vi "T1_viewer_gui.vi"() -> ()   [LabVIEW 2014]
uses:
  <vilib>/Analysis/NI_AALBase.lvlib
panel:
  in  "plots_tabs":enum32{"T1 curves", "Pulses", "Overlap pulses"}(tab)
  out "t1_curves":T1(graph)
  out "detections":u32[](graph)
  out "detections_norm":dbl[](graph)
  out "pulses":u32[][](graph)
  in  "show_all":bool
  in  "hide_all":bool
  out "snr_pulses":dbl
  out "mean_pulses":dbl format="%0.2f"
  in  "normalise_method":enum16{"No normalise", "Minimum", "Same pulse"}(ring)
  in  "save":bool
  in  "parameters":enum32{"No Selection", "uniform", "proposed"}(radio)=enum."uniform" caption="Parameters"
  in  "use_proposed_correction":bool
  in  "propose_rw":bool
  in  "propose_correction":bool
  in  "calc_parameters":bool
  in  "read_width_us":dbl
  in  "correction_us":dbl
  in  "compute_T1":bool
  in  "parameters":i32(listbox)
  out "progress":u8(slide) scale=0.0..100.0
  in  "plot_curves":bool
  in  "file_list":i32[](listbox)
  in  "files_folder":path
  in  "stop":bool
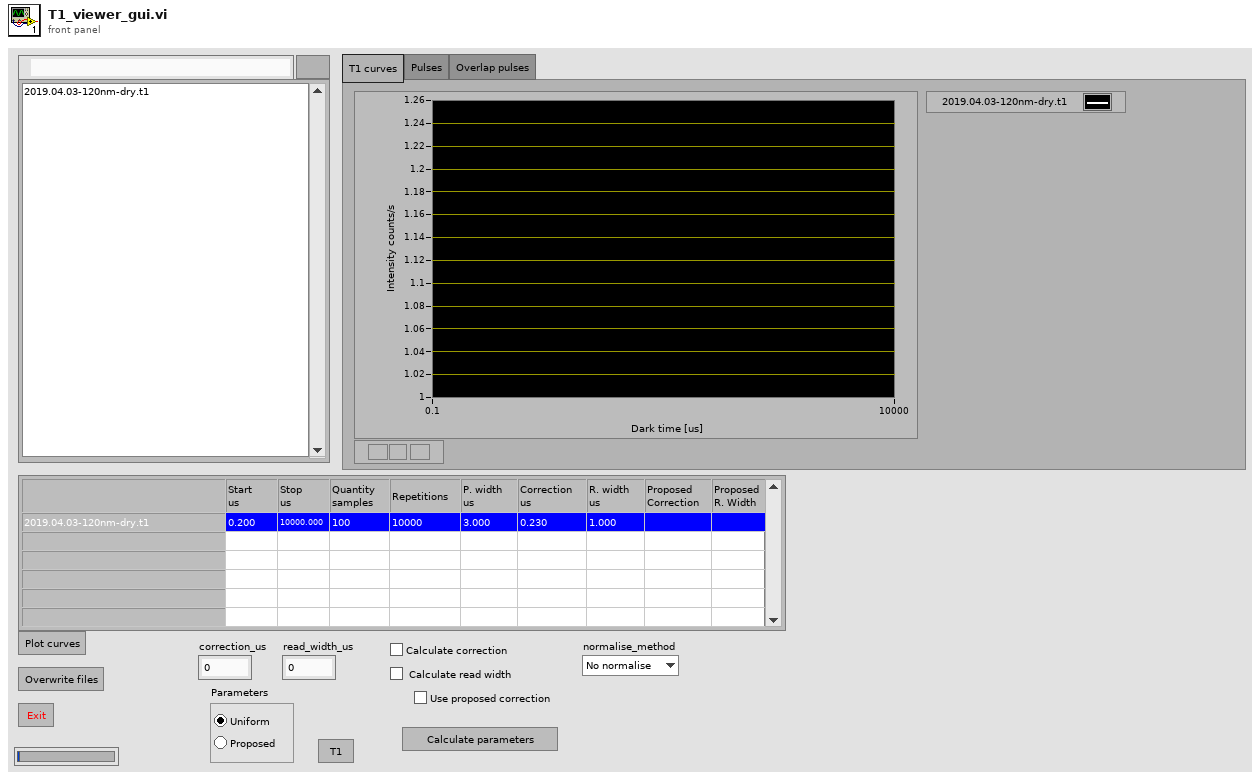
[diagram p1: front panel]
types:
  T1 = cluster{"dark_times_us":dbl[], "measured_signal":dbl[]}[]
  T2 = cluster{"dark_time_us":dbl[], "PL_signal":dbl[]}[]
  T3 = enum16{"standby", "plot", "fit", "compute_T1", "calc_correction"}
  T4 = enum16{"standby", "plot", "fit", "compute_T1", "calc_correction", "save"}
  T5 = enum16{"standby", "plot", "fit", "compute_T1", "calc_correction", "save", "plot_pulses"}
  T6 = cluster{"dark_times_us":dbl[], "measured_signal":dbl[]}
  T7 = cluster{"dark_times_us":dbl[], "pulse_width_us":dbl, "read_delay_us":dbl, "read_width_us":dbl, "repetitions":i32, "sampling_mode":enum16{"Normal", "Sweep"}, "correction_us":dbl}
  T8 = cluster{"dark_times":dbl[], "fitted_signal":dbl[]}
  T9 = cluster{"Ie":dbl, "Cm":dbl, "Tm":dbl, "C1":dbl, "T1":dbl, "mse":dbl}
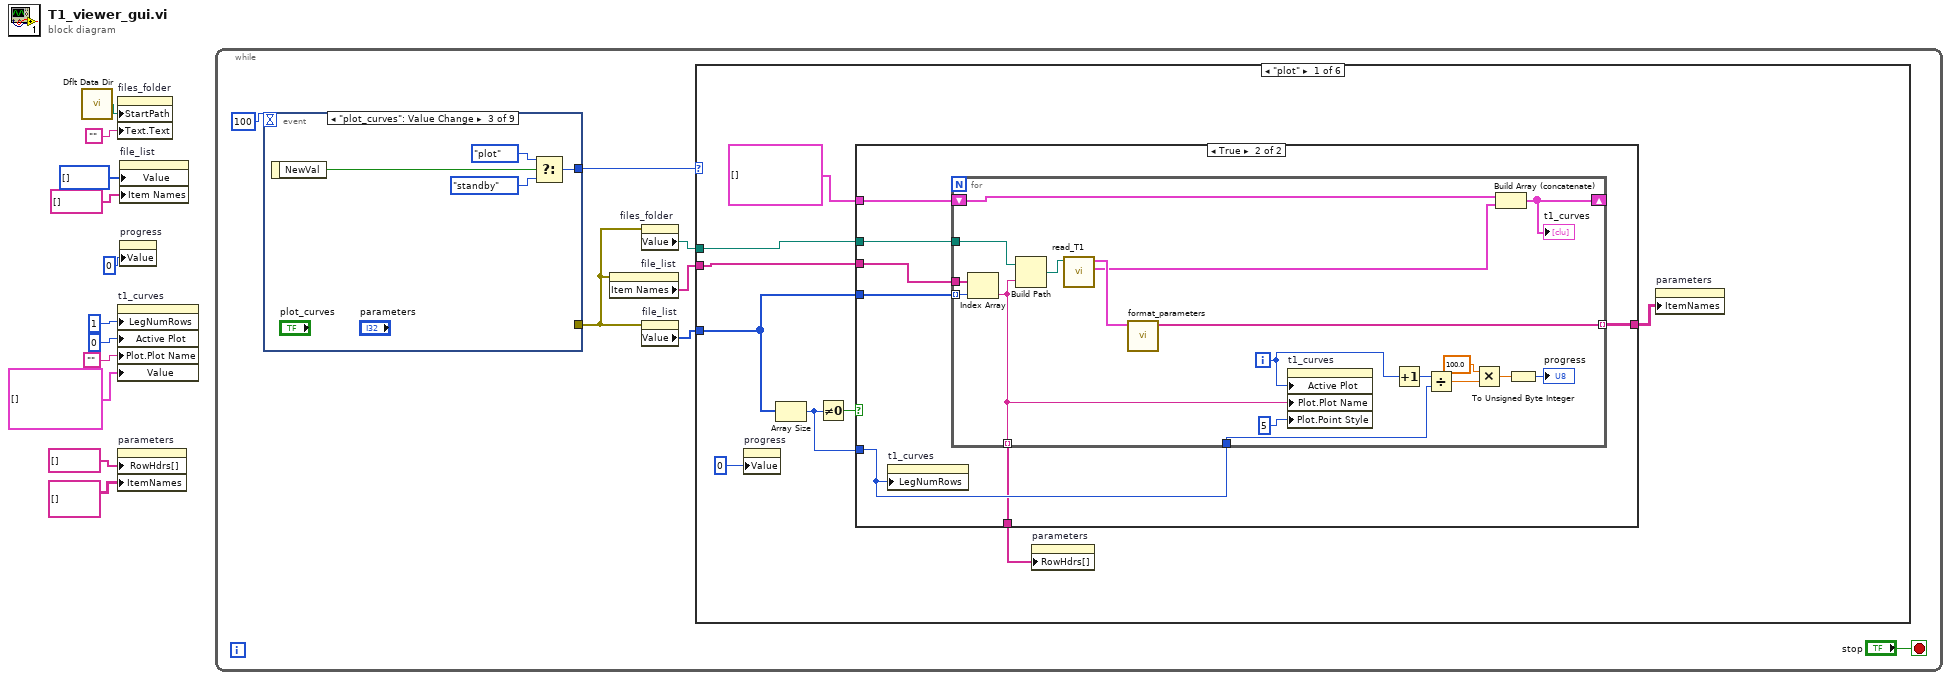
[diagram p0: block diagram]
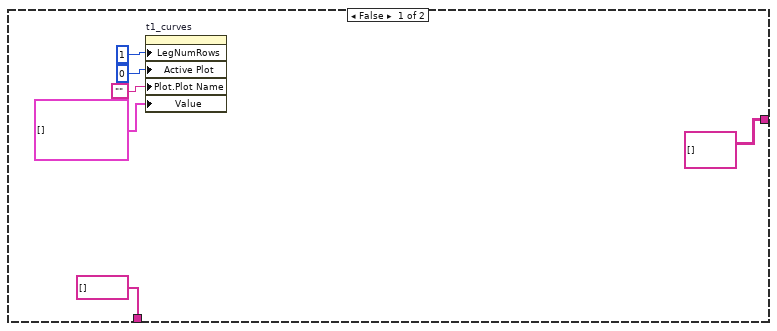
[diagram p2: hidden frame]
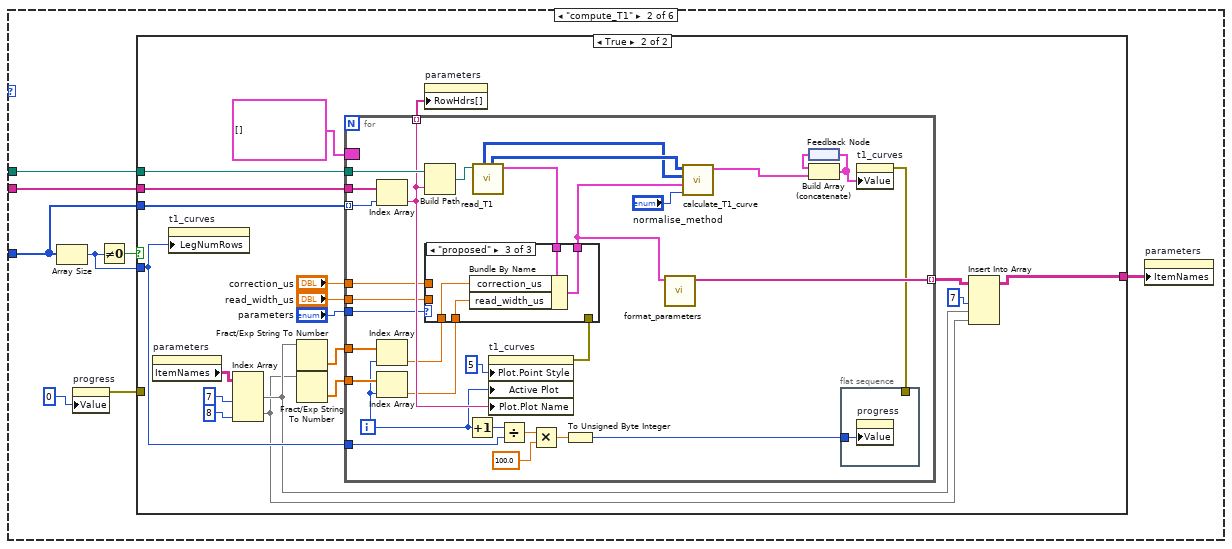
[diagram p3: hidden frame]
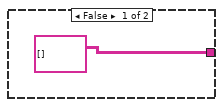
[diagram p4: hidden frame]
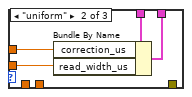
[diagram p6: hidden frame]
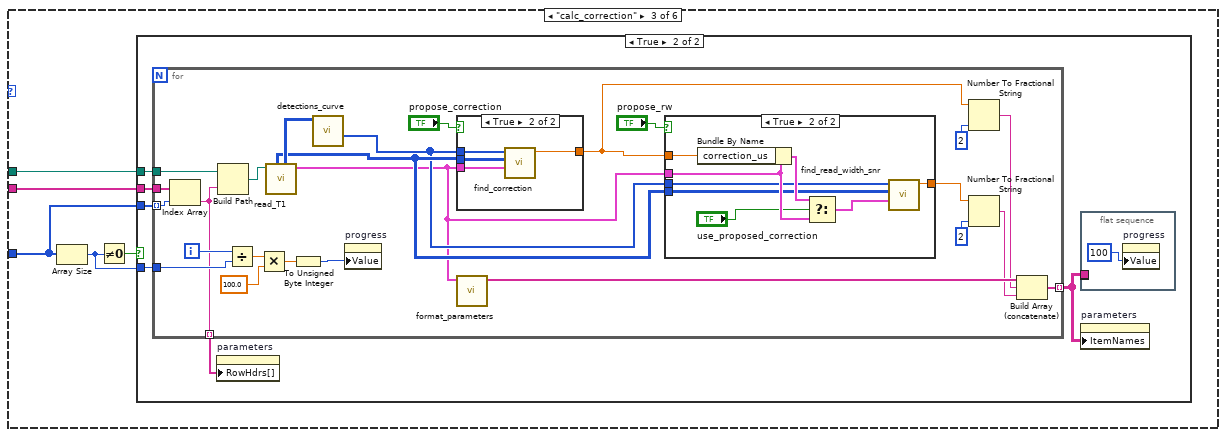
[diagram p7: hidden frame]
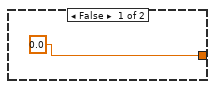
[diagram p9: hidden frame]
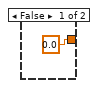
[diagram p10: hidden frame]
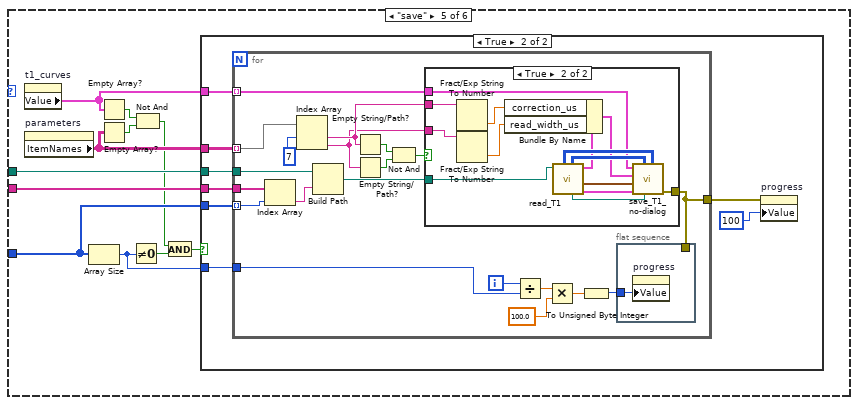
[diagram p12: hidden frame]
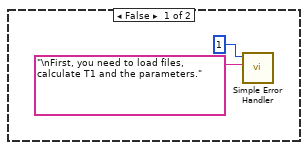
[diagram p13: hidden frame]
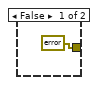
[diagram p14: hidden frame]
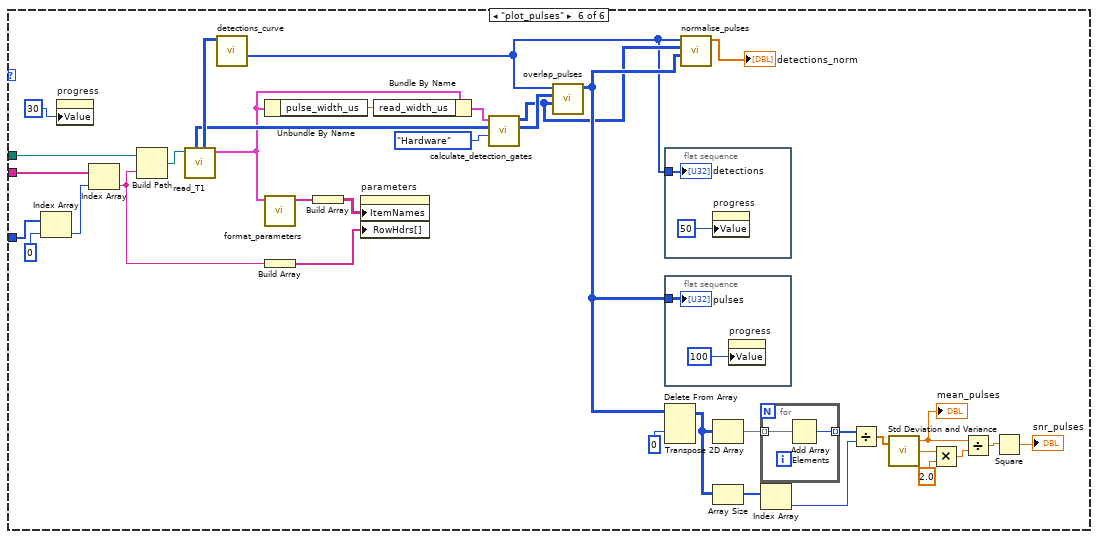
[diagram p15: hidden frame]
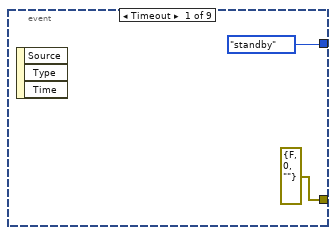
[diagram p16: hidden frame]
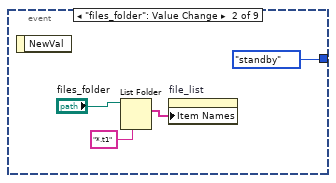
[diagram p17: hidden frame]
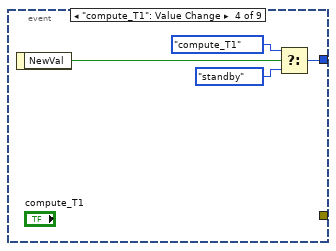
[diagram p18: hidden frame]
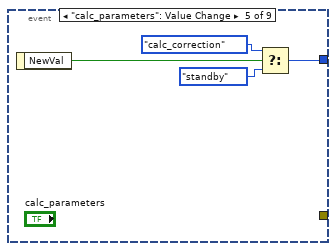
[diagram p19: hidden frame]
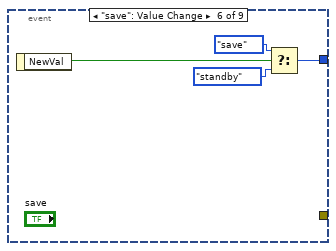
[diagram p20: hidden frame]
diagram:
  n1 = call <vilib>:"Dflt Data Dir.vi"() -> ("App:Default Data Directory"=w9:path)
  n2 = property on="files_folder" class="Path"("StartPath"=w9, "Text.Text"="") -> ()  [unwired: 2 in, 2 out]
  n3 = property on="t1_curves" class="XYGraph (strict)"("LegNumRows"=u32 1 ("Legend:Number of Rows"), "Active Plot"=u32 0, "Plot.Plot Name"="", "Value"=T1 [] ("t1_curves")) -> ()  [unwired: 2 in, 2 out]
  n4 = property on="parameters" class="MCListbox (strict)"("RowHdrs[]"=string[] [] ("Row Header Strings[]"), "ItemNames"=string[][] [] ("Item Names")) -> ()  [unwired: 2 in, 2 out]
  n5 = property on="file_list" class="LstBox (strict)"("Value"=i32[] [] ("file_list"), "Item Names"=string[] []) -> ()  [unwired: 2 in, 2 out]
  n6 = property on="progress" class="Slide (strict)"("Value"=u8 0 ("progress")) -> ()  [unwired: 2 in, 2 out]
  n7 = while {
    stop <- "stop" stop-if-true
    n8 = event shown="[2] \"plot_curves\": Value Change" {
      selector: _ -> [_ _ _ _ _ _ _ _ _]
      dyn-events: _ -> [_ _ _ _ _ _ _ _ _]
      timeout: 100 -> [_ _ _ _ _ _ _ _ _]
      tunnel: [enum16{"standby", "plot"}."standby" enum16{"standby", "plot"}."standby" w286 w291 w294 w298 T5."standby" T5."standby" w311] -> w16
      tunnel: [errorcluster {"status"=FALSE, "code"=0, "source"=""} ("error in (no error)") _ _ _ _ _ _ _ _] -> w12
      event Timeout {
        n9 = event-data() -> ()  [unwired: 1 in, 3 out]
      }
      event "files_folder": Value Change {
        n10 = event-data() -> ()  [unwired: 1 in, 1 out]
        n11 = List Folder(path="files_folder", pattern="*.t1") -> (filenames=w281:string[])  [unwired: 2 in, 3 out]
        n12 = property on="file_list" class="LstBox (strict)"("Item Names"=w281) -> ()  [unwired: 2 in, 2 out]
      }
      event "plot_curves": Value Change {
        n13 = event-data() -> ("NewVal"=w287:bool)  [unwired: 1 in]
        n14 = Select(t=enum16{"standby", "plot", "fit"}."plot", s=w287, f=enum16{"standby", "plot", "fit"}."standby") -> (s? t:f=w286:enum16{"standby", "plot", "fit"})
      }
      event "compute_T1": Value Change {
        n15 = event-data() -> ("NewVal"=w288:bool)  [unwired: 1 in]
        n16 = Select(t=enum16{"standby", "plot", "fit", "compute_T1"}."compute_T1", s=w288, f=enum16{"standby", "plot", "fit", "compute_T1"}."standby") -> (s? t:f=w291:enum16{"standby", "plot", "fit", "compute_T1"})
      }
      event "calc_parameters": Value Change {
        n17 = event-data() -> ("NewVal"=w292:bool)  [unwired: 1 in]
        n18 = Select(t=T3."calc_correction", s=w292, f=T3."standby") -> (s? t:f=w294:T3)
      }
      event "save": Value Change {
        n19 = event-data() -> ("NewVal"=w296:bool)  [unwired: 1 in]
        n20 = Select(t=T4."save", s=w296, f=T4."standby") -> (s? t:f=w298:T4)
      }
      event "hide_all": Value Change {
        n21 = event-data() -> ()  [unwired: 1 in, 1 out]
        n22 = while {
          i -> [w303]
          stop <- w301 stop-if-true
          n23 = property on="pulses" class="WFGraph (strict)"("Active Plot"=w303, "Plot.Visible?"=FALSE ("Plot.Visible")) -> (error out=w301:errorcluster)  [unwired: 2 in, 1 out]
        }
      }
      event "show_all": Value Change {
        n24 = event-data() -> ()  [unwired: 1 in, 1 out]
        n25 = while {
          i -> [w306]
          stop <- w307 stop-if-true
          n26 = property on="pulses" class="WFGraph (strict)"("Active Plot"=w306, "Plot.Visible?"=TRUE ("Plot.Visible")) -> (error out=w307:errorcluster)  [unwired: 2 in, 1 out]
        }
      }
      event "file_list": Value Change {
        n27 = event-data() -> ("NewVal"=w310:i32[])  [unwired: 1 in]
        n28 = Empty Array?(array=w310) -> (empty?=w309:bool)
        n29 = Not(x=w309) -> (.not. x?=w308:bool)
        n30 = case shown="True" w308 {
          tunnel: [T5."standby" w313] -> w311
          frame False {
          }
          frame True {
            n31 = case shown="\"T1 curves\", Default" "plots_tabs" {
              tunnel: [T5."standby" T5."plot_pulses" T5."plot_pulses"] -> w313
              frame "T1 curves", Default {
              }
              frame "Pulses" {
              }
              frame "Overlap pulses" {
              }
            }
          }
        }
      }
    }
    n32 = property on="file_list" class="LstBox (strict)"(error in=w12) -> ("Item Names"=w14:string[])  [unwired: 1 in, 2 out]
    n33 = property on="files_folder" class="Path"(error in=w12) -> ("Value"=w15:path)  [unwired: 1 in, 2 out]
    n34 = property on="file_list" class="LstBox (strict)"(error in=w12) -> ("Value"=w13:i32[])  [unwired: 1 in, 2 out]
    n35 = case shown="\"plot\"" w16 {
      tunnel: w15 -> [w19 w65 w132 _ w190 w271]
      tunnel: w14 -> [w20 w64 w131 _ w189 w270]
      tunnel: w13 -> [w21 w62 w129 _ w188 w258]
      frame "plot" {
        n36 = property on="progress" class="Slide (strict)"("Value"=u8 0 ("progress")) -> ()  [unwired: 2 in, 2 out]
        n37 = Array Size(array=w21) -> (size(s)=w26:i32)
        n38 = Not Equal To 0?(x=w26) -> (x != 0?=w27:bool)
        n39 = case shown="True" w27 {
          tunnel: w19 -> [_ w40]
          tunnel: w21 -> [_ w39]
          tunnel: w26 -> [_ w38]
          tunnel: T1 [] ("t1_curves") -> [_ w37]
          tunnel: w20 -> [_ w36]
          tunnel: [string[] [] w35] -> w23
          tunnel: [string[][] [] ("parameters") w34] -> w22
          frame False {
            n40 = property on="t1_curves" class="XYGraph (strict)"("LegNumRows"=u32 1 ("Legend:Number of Rows"), "Active Plot"=u32 0, "Plot.Plot Name"="", "Value"=T1 [] ("t1_curves")) -> ()  [unwired: 2 in, 2 out]
          }
          frame True {
            n41 = property on="t1_curves" class="XYGraph (strict)"("LegNumRows"=w38) -> ()  [unwired: 2 in, 2 out]
            n42 = for {
              tunnel: w39 -> [w58] mode=indexing
              tunnel: w40 -> [w56]
              tunnel: w38 -> [w43]
              shift-right: [w54] -> _
              shift-left: w37 -> [w42]
              tunnel: w36 -> [w53]
              tunnel: [w52] -> w35 mode=indexing
              tunnel: [w50] -> w34 mode=indexing
              i -> [w44]
              n43 = Index Array(array=w53, index=w58) -> (element=w52:string)
              n44 = Build Path(base path=w56, name or relative path=w52) -> (appended path=w57:path)
              n45 = call "read_T1.vi"("file_path"=w57) -> ("T1_curve"=w41:T6, "T1_parameters"=w51:T7)  [unwired: 4 in, 5 out]
              n46 = call "format_parameters.vi"("T1_parameters"=w51) -> ("parameters_strg"=w50:string[])  [unwired: 9 in, 1 out]
              n47 = property on="t1_curves" class="XYGraph (strict)"("Active Plot"=w44, "Plot.Plot Name"=w52, "Plot.Point Style"=u8 5) -> ()  [unwired: 2 in, 2 out]
              n48 = Increment(x=w44) -> (x+1=w49:i32)
              n49 = Divide(x=w49, y=w43) -> (x/y=w47:dbl)
              n50 = Multiply(x=100.0, y=w47) -> (x*y=w46:dbl)
              n51 = Build Array (concatenate)(w42, w41) -> (w54:T1)
              "t1_curves" <- w54
              n52 = To Unsigned Byte Integer(number=w46) -> (unsigned 8bit integer=→"progress":u8)
            }
          }
        }
        n53 = property on="parameters" class="MCListbox (strict)"("RowHdrs[]"=w23) -> ()  [unwired: 2 in, 2 out]
        n54 = property on="parameters" class="MCListbox (strict)"("ItemNames"=w22) -> ()  [unwired: 2 in, 2 out]
      }
      frame "compute_T1" {
        n55 = Array Size(array=w62) -> (size(s)=w63:i32)
        n56 = property on="progress" class="Slide (strict)"("Value"=u8 0 ("progress")) -> (error out=w59:errorcluster)  [unwired: 2 in, 1 out]
        n57 = Not Equal To 0?(x=w63) -> (x != 0?=w66:bool)
        n58 = case shown="True" w66 {
          tunnel: w65 -> [_ w86]
          tunnel: w64 -> [_ w85]
          tunnel: w62 -> [_ w84]
          tunnel: [string[][] [] ("parameters") w75] -> w60
          tunnel: w63 -> [_ w82]
          tunnel: w59 -> [_ _]
          frame False {
          }
          frame True {
            n59 = property on="parameters" class="MCListbox (strict)"() -> ("ItemNames"=w77:string[][])  [unwired: 2 in, 2 out]
            n60 = property on="t1_curves" class="XYGraph (strict)"("LegNumRows"=w82) -> ()  [unwired: 2 in, 2 out]
            n61 = Index Array(array=w77, index (col) #1=7 ("index (row)"), index (col) #2=8 ("index (row)")) -> (element #1=w73:string[], element #2=w71:string[])  [unwired: 2 in]
            n62 = Fract/Exp String To Number(string=w73) -> (number=w72:dbl[])  [unwired: 3 in, 1 out]
            n63 = Fract/Exp String To Number(string=w71) -> (number=w70:dbl[])  [unwired: 3 in, 1 out]
            n64 = for {
              tunnel: w86 -> [w117]
              tunnel: w85 -> [w113]
              tunnel: "correction_us" -> [w97]
              tunnel: "read_width_us" -> [w96]
              border: T2 [] -> [_]
              tunnel: w84 -> [w114] mode=indexing
              tunnel: [w111] -> w76 mode=indexing
              tunnel: w82 -> [w109]
              tunnel: [w103] -> w83 mode=indexing
              tunnel: w72 -> [w94]
              tunnel: w70 -> [w92]
              tunnel: "parameters" -> [w95]
              i -> [w90]
              n65 = Index Array(array=w113, index=w114) -> (element=w103:string)
              n66 = Index Array(array=w94, index=w90) -> (element=w93:dbl)
              n67 = Index Array(array=w92, index=w90) -> (element=w91:dbl)
              n68 = Build Path(base path=w117, name or relative path=w103) -> (appended path=w116:path)
              n69 = Increment(x=w90) -> (x+1=w110:i32)
              n70 = call "read_T1.vi"("file_path"=w116) -> ("T1_parameters"=w101:T7, "timetags"=w102:u32[][], "triggers"=w100:u32[][])  [unwired: 4 in, 4 out]
              n71 = property on="t1_curves" class="XYGraph (strict)"("Plot.Point Style"=u8 5, "Active Plot"=w90, "Plot.Plot Name"=w103) -> (error out=w104:errorcluster)  [unwired: 2 in, 1 out]
              n72 = case shown="\"proposed\"" w95 {
                tunnel: [w119 w120 w127] -> w112
                tunnel: w101 -> [w119 w123 w126]
                tunnel: w96 -> [_ w122 _]
                tunnel: w97 -> [_ w121 _]
                tunnel: w104 -> [_ _ _]
                tunnel: w91 -> [_ _ w125]
                tunnel: w93 -> [_ _ w124]
                frame "No Selection", Default {
                }
                frame "uniform" {
                  n73 = Bundle By Name(cluster=w123, "correction_us"=w121, "read_width_us"=w122) -> (w120:T7)
                }
                frame "proposed" {
                  n74 = Bundle By Name(cluster=w126, "correction_us"=w124, "read_width_us"=w125) -> (w127:T7)
                }
              }
              n75 = Divide(x=w110, y=w109) -> (x/y=w108:dbl)
              n76 = Multiply(x=w108, y=100.0) -> (x*y=w106:dbl)
              n77 = To Unsigned Byte Integer(number=w106) -> (unsigned 8bit integer=w99:u8)
              n78 = call "format_parameters.vi"("T1_parameters"=w112) -> ("parameters_strg"=w111:string[])  [unwired: 9 in, 1 out]
              n79 = call "calculate_T1_curve.vi"("normalise"="normalise_method", "T1_parameters"=w112, "triggers"=w100, "timetags"=w102) -> ("T1_curve_out"=w89:cluster{"dark_time_us":dbl[], "PL_signal":dbl[]})  [unwired: 7 in]
              n80 = feedback #1() -> (w115:T2)
              n81 = Build Array (concatenate)(w115, w89) -> (w88:T2)
              n82 = feedback-in #1(w88) -> ()
              n83 = flat-sequence {
                tunnel: w99 -> [w118]
                tunnel: w98 -> [_]
                frame #0 {
                  n84 = property on="progress" class="Slide (strict)"("Value"=w118) -> ()  [unwired: 2 in, 2 out]
                }
              }
              n85 = property on="t1_curves" class="XYGraph (strict)"("Value"=w88) -> (error out=w98:errorcluster)  [unwired: 2 in, 1 out]
            }
            n86 = property on="parameters" class="MCListbox (strict)"("RowHdrs[]"=w83) -> ()  [unwired: 2 in, 2 out]
            n87 = Insert Into Array(array=w76, index (col)=7 ("disabled index (col)"), new element #1=w73, new element #2=w71) -> (w75:string[][])  [unwired: 1 in]
          }
        }
        n88 = property on="parameters" class="MCListbox (strict)"("ItemNames"=w60) -> ()  [unwired: 2 in, 2 out]
      }
      frame "calc_correction" {
        n89 = Array Size(array=w129) -> (size(s)=w128:i32)
        n90 = Not Equal To 0?(x=w128) -> (x != 0?=w130:bool)
        n91 = case shown="True" w130 {
          tunnel: w132 -> [_ w138]
          tunnel: w131 -> [_ w137]
          tunnel: w129 -> [_ w136]
          tunnel: w128 -> [_ w135]
          frame False {
          }
          frame True {
            n92 = for {
              tunnel: w138 -> [w165]
              tunnel: w137 -> [w162]
              tunnel: w136 -> [w163] mode=indexing
              tunnel: w135 -> [w161]
              tunnel: [w149] -> w133 mode=indexing
              tunnel: [w141] -> w134 mode=indexing
              i -> [w142]
              n93 = Index Array(array=w162, index=w163) -> (element=w141:string)
              n94 = Build Path(base path=w165, name or relative path=w141) -> (appended path=w164:path)
              n95 = Divide(x=w142, y=w161) -> (x/y=w160:dbl)
              n96 = Multiply(x=w160, y=100.0) -> (x*y=w158:dbl)
              n97 = call "read_T1.vi"("file_path"=w164) -> ("T1_parameters"=w151:T7, "timetags"=w156:u32[][], "triggers"=w153:u32[][])  [unwired: 4 in, 4 out]
              n98 = To Unsigned Byte Integer(number=w158) -> (unsigned 8bit integer=w157:u8)
              n99 = call "detections_curve.vi"("timetags"=w156) -> ("detections"=w152:u32[])  [unwired: 10 in]
              n100 = property on="progress" class="Slide (strict)"("Value"=w157) -> ()  [unwired: 2 in, 2 out]
              n101 = case shown="True" "propose_correction" {
                tunnel: [0.0 ("shift_us") w179] -> w148
                tunnel: w152 -> [_ w178]
                tunnel: w153 -> [_ w177]
                tunnel: w151 -> [_ w176]
                frame False {
                }
                frame True {
                  n102 = call "find_correction.vi"("T1_parameters"=w176, "triggers"=w177, "detections"=w178) -> ("shift_us"=w179:dbl)  [unwired: 8 in]
                }
              }
              n103 = call "format_parameters.vi"("T1_parameters"=w151) -> ("parameters_strg"=w150:string[])  [unwired: 9 in, 1 out]
              n104 = case shown="True" "propose_rw" {
                tunnel: [0.0 ("proposed_read_width_us") w167] -> w145
                tunnel: w151 -> [_ w172]
                tunnel: w148 -> [_ w174]
                tunnel: w153 -> [_ w169]
                tunnel: w152 -> [_ w170]
                frame False {
                }
                frame True {
                  n105 = Bundle By Name(cluster=w172, "correction_us"=w174) -> (w173:T7)
                  n106 = Select(t=w173, s="use_proposed_correction", f=w172) -> (s? t:f=w168:T7)
                  n107 = call "find_read_width_snr.vi"("T1_parameters"=w168, "triggers"=w169, "detections"=w170) -> ("read_width_us"=w167:dbl)  [unwired: 8 in]
                }
              }
              n108 = Number To Fractional String(number=w148, precision (6)=i16 2) -> (F-format string=w144:string)  [unwired: 2 in]
              n109 = Number To Fractional String(number=w145, precision (6)=i16 2) -> (F-format string=w143:string)  [unwired: 2 in]
              n110 = Build Array (concatenate)(w150, w144, w143) -> (w149:string[])
            }
            n111 = property on="parameters" class="MCListbox (strict)"("RowHdrs[]"=w134) -> ()  [unwired: 2 in, 2 out]
            n112 = flat-sequence {
              tunnel: [w139] -> _
              tunnel: w133 -> [w139]
              frame #0 {
                n113 = property on="progress" class="Slide (strict)"("Value"=u8 100 ("progress")) -> ()  [unwired: 2 in, 2 out]
              }
            }
            n114 = property on="parameters" class="MCListbox (strict)"("ItemNames"=w133) -> ()  [unwired: 2 in, 2 out]
          }
        }
      }
      frame "standby", Default {
      }
      frame "save" {
        n115 = property on="t1_curves" class="XYGraph (strict)"() -> ("Value"=w186:T1)  [unwired: 2 in, 2 out]
        n116 = property on="parameters" class="MCListbox (strict)"() -> ("ItemNames"=w185:string[][])  [unwired: 2 in, 2 out]
        n117 = Array Size(array=w188) -> (size(s)=w187:i32)
        n118 = Empty Array?(array=w186) -> (empty?=w184:bool)
        n119 = Empty Array?(array=w185) -> (empty?=w183:bool)
        n120 = Not Equal To 0?(x=w187) -> (x != 0?=w180:bool)
        n121 = Not And(1:w183, 2:w184) -> (0:w181:bool)
        n122 = And(x=w181, y=w180) -> (x .and. y?=w182:bool)
        n123 = case shown="True" w182 {
          tunnel: w190 -> [_ w200]
          tunnel: w189 -> [_ w199]
          tunnel: w188 -> [_ w198]
          tunnel: w187 -> [_ w197]
          tunnel: w185 -> [_ w196]
          tunnel: w186 -> [_ w195]
          frame False {
            n124 = call <vilib>:"Simple Error Handler.vi"("error code (no error:0)"=1, "error source (\" \")"="\nFirst, you need to load files, calculate T1 and the parameters." ("error source (\" \")")) -> ()  [unwired: 3 in, 5 out]
          }
          frame True {
            n125 = for {
              tunnel: w200 -> [w220]
              tunnel: w199 -> [w218]
              tunnel: w198 -> [w219] mode=indexing
              tunnel: w197 -> [w217]
              tunnel: w196 -> [w210] mode=indexing
              tunnel: w195 -> [w203] mode=indexing
              tunnel: [w201] -> w193
              i -> [w213]
              n126 = Index Array(array=w218, index=w219) -> (element=w212:string)
              n127 = Index Array(array=w210, index #1=7 ("index")) -> (element #1=w206:string, element #2=w204:string)  [unwired: 1 in]
              n128 = Build Path(base path=w220, name or relative path=w212) -> (appended path=w205:path)
              n129 = Empty String/Path?(string/path=w206) -> (empty?=w209:bool)
              n130 = Empty String/Path?(string/path=w204) -> (empty?=w208:bool)
              n131 = Not And(1:w208, 2:w209) -> (0:w207:bool)
              n132 = case shown="True" w207 {
                tunnel: w206 -> [_ w234]
                tunnel: w205 -> [_ w226]
                tunnel: w204 -> [_ w225]
                tunnel: w203 -> [_ w224]
                tunnel: [errorcluster {"status"=FALSE, "code"=0, "source"=""} ("error out") w223] -> w201
                frame False {
                }
                frame True {
                  n133 = Fract/Exp String To Number(string=w234) -> (number=w235:dbl)  [unwired: 3 in, 1 out]
                  n134 = Fract/Exp String To Number(string=w225) -> (number=w236:dbl)  [unwired: 3 in, 1 out]
                  n135 = call "read_T1.vi"("file_path"=w226) -> ("fitted_signal"=w232:T8, "fit_parameters"=w233:T9, "T1_parameters"=w227:T7, "file_path"=w231:path, "timetags"=w229:u32[][], "triggers"=w230:u32[][])  [unwired: 4 in, 1 out]
                  n136 = Bundle By Name(cluster=w227, "correction_us"=w235, "read_width_us"=w236) -> (w228:T7)
                  n137 = call "save_T1_no-dialog.vi"("triggers"=w230, "file_path"=w231, "timetags"=w229, "fitted_signal_in"=w232, "fit_parameters"=w233, "T1_parameters"=w228, "T1_curve_in"=w224) -> ("error out"=w223:errorcluster)  [unwired: 4 in]
                }
              }
              n138 = Divide(x=w213, y=w217) -> (x/y=w216:dbl)
              n139 = Multiply(x=w216, y=100.0) -> (x*y=w214:dbl)
              n140 = To Unsigned Byte Integer(number=w214) -> (unsigned 8bit integer=w202:u8)
              n141 = flat-sequence {
                tunnel: w202 -> [w221]
                tunnel: w201 -> [_]
                frame #0 {
                  n142 = property on="progress" class="Slide (strict)"("Value"=w221) -> ()  [unwired: 2 in, 2 out]
                }
              }
            }
            n143 = property on="progress" class="Slide (strict)"(error in=w193, "Value"=u8 100 ("progress")) -> ()  [unwired: 1 in, 2 out]
          }
        }
      }
      frame "plot_pulses" {
        n144 = Index Array(array=w258, index=0) -> (element=w259:i32)
        n145 = property on="progress" class="Slide (strict)"("Value"=u8 30 ("progress")) -> ()  [unwired: 2 in, 2 out]
        n146 = Index Array(array=w270, index=w259) -> (element=w264:string)
        n147 = Build Path(base path=w271, name or relative path=w264) -> (appended path=w269:path)
        n148 = call "read_T1.vi"("file_path"=w269) -> ("T1_parameters"=w244:T7, "timetags"=w268:u32[][], "triggers"=w267:u32[][])  [unwired: 4 in, 4 out]
        n149 = call "detections_curve.vi"("timetags"=w268) -> ("detections"=w238:u32[])  [unwired: 10 in]
        n150 = Unbundle By Name(w244) -> ("pulse_width_us"=w243:dbl)
        n151 = call "format_parameters.vi"("T1_parameters"=w244) -> ("parameters_strg"=w266:string[])  [unwired: 9 in, 1 out]
        n152 = Build Array(w264) -> (w263:string[])
        n153 = Build Array(w266) -> (w265:string[][])
        n154 = property on="parameters" class="MCListbox (strict)"("ItemNames"=w265, "RowHdrs[]"=w263) -> ()  [unwired: 2 in, 2 out]
        n155 = Bundle By Name(cluster=w244, "read_width_us"=w243) -> (w242:T7)
        n156 = call "calculate_detection_gates.vi"("gates_calculation"=enum16{"Software", "Hardware"}."Hardware", "triggers"=w267, "T1_parameters"=w242) -> ("start_read"=w262:u32[][], "stop_read"=w239:u32[][])  [unwired: 7 in]
        n157 = call "overlap_pulses.vi"("stop_read"=w239, "start_read"=w262, "detections"=w238) -> ("pulses"=w240:u32[][])  [unwired: 8 in]
        n158 = flat-sequence {
          tunnel: w238 -> [w276]
          frame #0 {
            n159 = property on="progress" class="Slide (strict)"("Value"=u8 50 ("progress")) -> ()  [unwired: 2 in, 2 out]
            "detections" <- w276
          }
        }
        n160 = flat-sequence {
          tunnel: w240 -> [w274]
          frame #0 {
            n161 = property on="progress" class="Slide (strict)"("Value"=u8 100 ("progress")) -> ()  [unwired: 2 in, 2 out]
            "pulses" <- w274
          }
        }
        n162 = Delete From Array(array=w240, index (row)=0) -> (array with subset deleted=w254:u32[][])  [unwired: 2 in, 1 out]
        n163 = call "normalise_pulses.vi"("pulses"=w240, "stop_read"=w239, "detections"=w238) -> ("detections_normalised"=→"detections_norm":dbl[])  [unwired: 8 in]
        n164 = Transpose 2D Array(2D array=w254) -> (transposed array=w255:u32[][])
        n165 = Array Size(array=w254) -> (size(s)=w253:i32[])
        n166 = for {
          tunnel: w255 -> [w273] mode=indexing
          tunnel: [w272] -> w256 mode=indexing
          n167 = Add Array Elements(numeric array=w273) -> (sum=w272:u32)
        }
        n168 = Index Array(array=w253) -> (element=w252:i32)  [unwired: 1 in]
        n169 = Divide(x=w256, y=w252) -> (x/y=w245:dbl[])
        n170 = call <vilib>:"Std Deviation and Variance.vi"("X"=w245) -> ("mean"=w251:dbl, "standard deviation"=w249:dbl)  [unwired: 1 in, 1 out]
        "mean_pulses" <- w251
        n171 = Multiply(x=w249, y=2.0 ("x")) -> (x*y=w248:dbl)
        n172 = Divide(x=w251, y=w248) -> (x/y=w247:dbl)
        n173 = Square(x=w247) -> (x^2=→"snr_pulses":dbl)
      }
    }
  }
